vi "Create DVR API for Class Method.vi"(6 "DVR API Suffix":string=" API", 8 "error in (no error)":errorcluster, 9 "Class DVR Control File Path":path, 10 "DVR API Directory Path":path, 11 "Class Method Path":path) -> (0 "error out":errorcluster, 3 "DVR VI Path":path)   [LabVIEW 2016, in "SLL Scripting.lvlib" / "SLL Class DVR API Generator.lvlib"]
uses:
  SLL Class DVR API Generator.lvlib
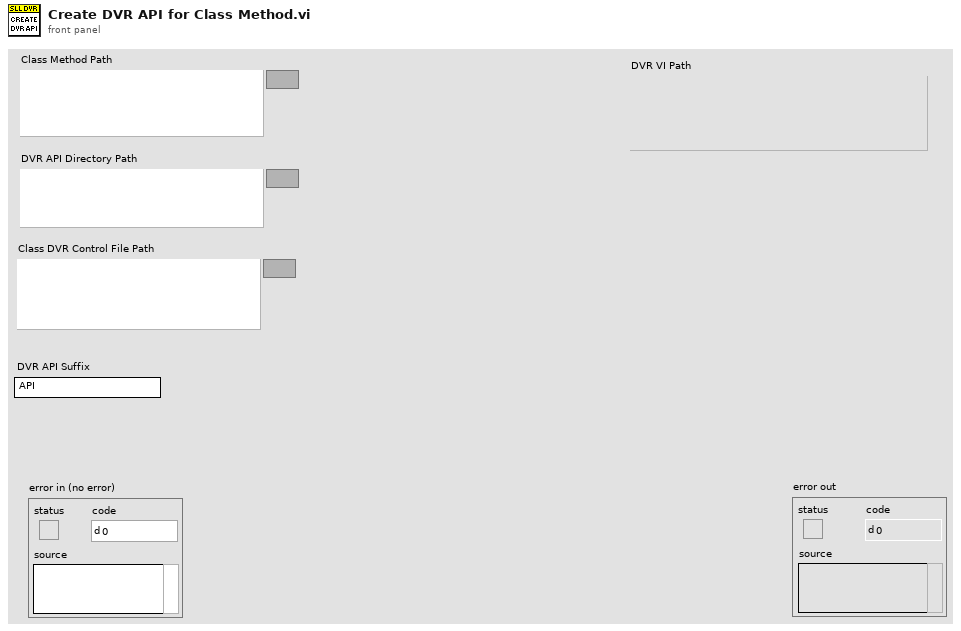
[diagram p1: front panel]
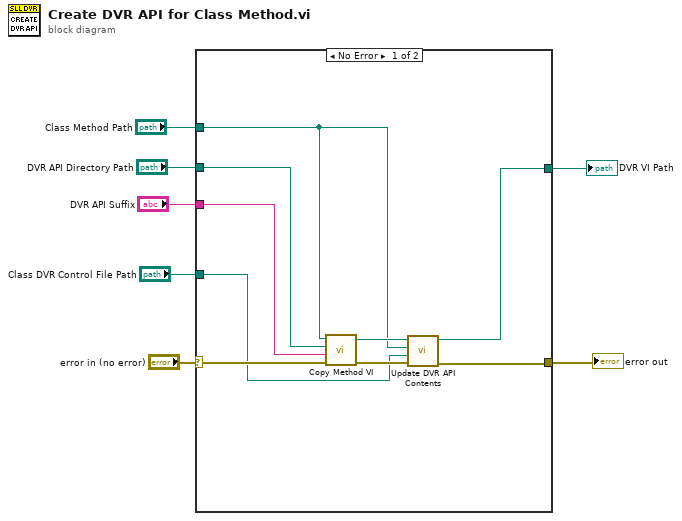
[diagram p0: block diagram]
diagram:
  n1 = case shown="No Error" "error in (no error)" {
    selector: "error in (no error)" -> [w14 w17]
    tunnel: "Class Method Path" -> [w11 _]
    tunnel: "DVR API Directory Path" -> [w16 _]
    tunnel: "DVR API Suffix" -> [w15 _]
    tunnel: [w10 w17] -> w3
    tunnel: "Class DVR Control File Path" -> [w9 _]
    tunnel: [w8 _] -> w1
    frame No Error {
      n2 = call "Copy Method VI.vi"("error in (no error)"=w14, "DVR API Suffix"=w15, "DVR API Directory Path"=w16, "Class Method Path"=w11) -> ("error out"=w13:errorcluster, "DVR Method Path Out"=w12:path)  [unwired: 6 in]
      n3 = call "Update DVR API Contents.vi"("error in (no error)"=w13, "Class DVR Control File Path"=w9, "Method Path"=w11, "DVR API Path"=w12) -> ("error out"=w10:errorcluster, "DVR VI Path"=w8:path)  [unwired: 6 in]
    }
    frame Error {
    }
  }
  "error out" <- w3
  "DVR VI Path" <- w1
